vi "picoquant_initialize_acq_mode.vi"(8 "error in (no error)":errorcluster, 11 "hydraharp in":refnum<class "hydraharp.lvclass">) -> (0 "error out":errorcluster, 3 "hydraharp out":refnum<class "hydraharp.lvclass">)   [LabVIEW 2015, in "hydraharp.lvclass"]
uses:
  hydraharp.lvclass
  hydraharp.lvclass/hydraharp.ctl
  hhlib.dll
panel:
  out "version":u8[](array[numeric])
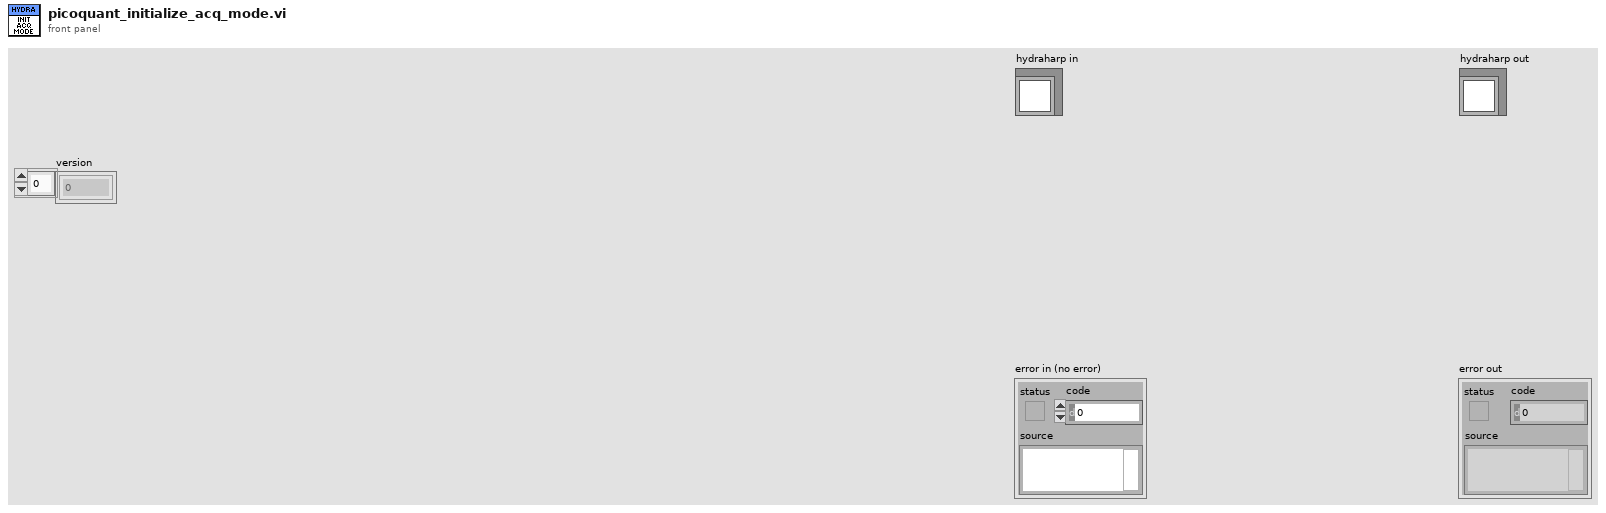
[diagram p1: front panel]
types:
  T1 = typedef "hpanel_acq_modes.ctl" = u16
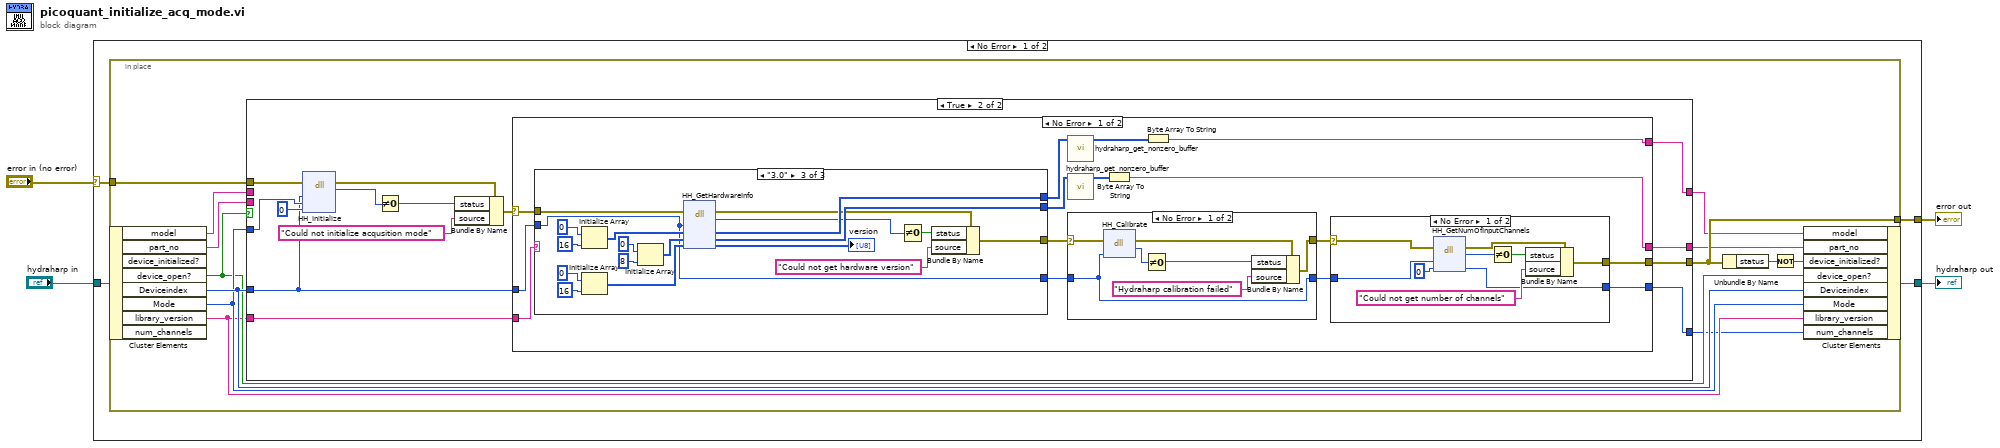
[diagram p0: block diagram]
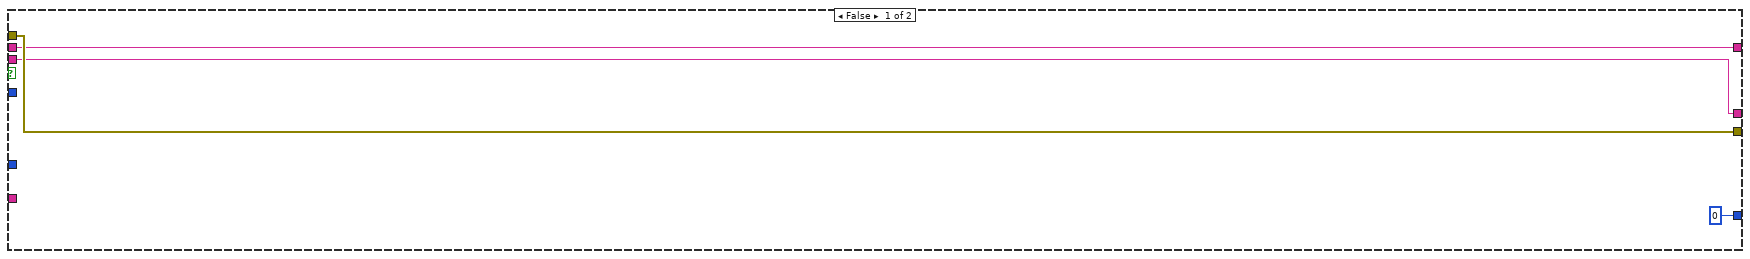
[diagram p2: hidden frame]
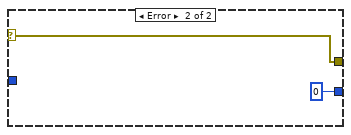
[diagram p3: hidden frame]
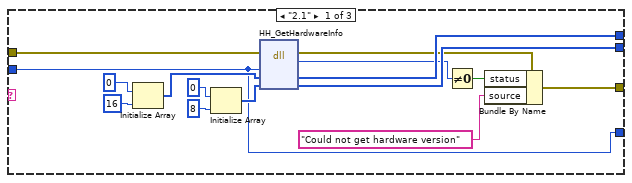
[diagram p5: hidden frame]
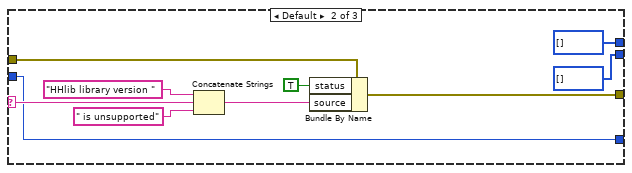
[diagram p6: hidden frame]
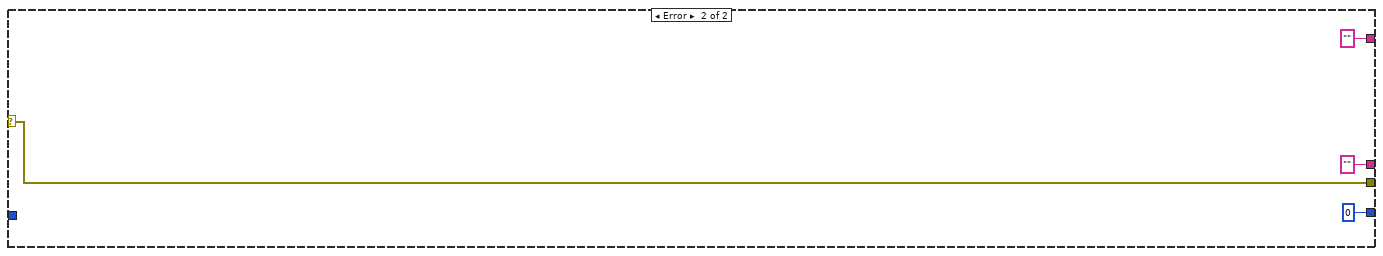
[diagram p7: hidden frame]
diagram:
  n1 = case shown="No Error" "error in (no error)" {
    selector: "error in (no error)" -> [w7 w124]
    tunnel: [w6 w124] -> w1
    tunnel: [w5 w123] -> w2
    tunnel: "hydraharp in" -> [w8 w123]
    frame No Error {
      n2 = in-place {
        in-place-border: w7 -> [w21]
        in-place-border: [w17] -> w6
        n3 = in-place-cluster #1(w8) -> ("model"=w12:string, "part_no"=w11:string, "device_open?"=w18:bool, "Deviceindex"=w20:i32, "Mode"=w19:T1, "library_version"=w10:string)  [unwired: 2 out]
        n4 = case shown="True" w18 {
          tunnel: w21 -> [w25 w39]
          tunnel: [w25 w36] -> w17
          tunnel: w20 -> [_ w35]
          tunnel: w19 -> [_ w37]
          tunnel: [w24 w34] -> w14
          tunnel: [w23 w33] -> w13
          tunnel: w12 -> [w24 _]
          tunnel: w11 -> [w23 _]
          tunnel: w10 -> [_ w32]
          tunnel: [0 ("num_channels") w26] -> w9
          frame False {
          }
          frame True {
            n5 = dll-call lib="hhlib.dll" fn="HH_Initialize"(error in=w39, "devidx"=w35, "mode"=w37, "refsrc"=0) -> (error out=w30:errorcluster, w31:i32)  [unwired: 5 in, 1 out]
            n6 = Not Equal To 0?(x=w31) -> (x != 0?=w29:bool)
            n7 = Bundle By Name(cluster=w30, "status"=w29, "source"="Could not initialize acqusition mode") -> (w27:errorcluster)
            n8 = case shown="No Error" w27 {
              selector: w27 -> [w44 w120]
              tunnel: [w42 w120] -> w36
              tunnel: w35 -> [w54 _]
              tunnel: [w48 "" ("string")] -> w34
              tunnel: [w47 "" ("string")] -> w33
              tunnel: w32 -> [w46 _]
              tunnel: [w40 0 ("num_channels")] -> w26
              frame No Error {
                n9 = case shown="\"3.0\"" w46 {
                  selector: w46 -> [_ w96 _]
                  tunnel: w44 -> [w89 w94 w118]
                  tunnel: w54 -> [w80 w90 w105]
                  tunnel: [w77 w93 w100] -> w53
                  tunnel: [w82 u8[] [] ("Model") w111] -> w52
                  tunnel: [w81 u8[] [] ("Partno") w110] -> w51
                  tunnel: [w80 w90 w105] -> w45
                  frame "2.1" {
                    n10 = Initialize Array(u8 0 ("element"), 16 ("dimension size")) -> (w86:u8[])
                    n11 = Initialize Array(u8 0 ("element"), 8 ("dimension size")) -> (w83:u8[])
                    n12 = dll-call lib="hhlib.dll" fn="HH_GetHardwareInfo" label="HH_GetHardwareVersion"(error in=w89, "devidx"=w80, "Model"=w86, "Partno"=w83) -> (error out=w78:errorcluster, "return type"=w76:i32, "Model"=w82:u8[], "Partno"=w81:u8[])  [unwired: 3 in, 1 out]
                    n13 = Not Equal To 0?(x=w76) -> (x != 0?=w75:bool)
                    n14 = Bundle By Name(cluster=w78, "status"=w75, "source"="Could not get hardware version") -> (w77:errorcluster)
                  }
                  frame Default {
                    n15 = Concatenate Strings("HHlib library version " ("string"), w96, " is unsupported" ("string")) -> (w91:string)
                    n16 = Bundle By Name(cluster=w94, "status"=TRUE, "source"=w91) -> (w93:errorcluster)
                  }
                  frame "3.0" {
                    n17 = Initialize Array(u8 0 ("element"), 16 ("dimension size")) -> (w115:u8[])
                    n18 = Initialize Array(u8 0 ("element"), 16 ("dimension size")) -> (w107:u8[])
                    n19 = Initialize Array(u8 0 ("element"), 8 ("dimension size")) -> (w112:u8[])
                    n20 = dll-call lib="hhlib.dll" fn="HH_GetHardwareInfo" label="HH_GetHardwareVersion"(error in=w118, "devidx"=w105, "Model"=w115, "Partno"=w112, "version"=w107) -> (error out=w103:errorcluster, "return type"=w104:i32, "Model"=w111:u8[], "Partno"=w110:u8[], "version"=→"version":u8[])  [unwired: 3 in, 1 out]
                    n21 = Not Equal To 0?(x=w104) -> (x != 0?=w102:bool)
                    n22 = Bundle By Name(cluster=w103, "status"=w102, "source"="Could not get hardware version") -> (w100:errorcluster)
                  }
                }
                n23 = call "hydraharp_get_nonzero_buffer.vi"("buffer"=w52) -> ("subarray"=w49:u8[])  [unwired: 10 in]
                n24 = call "hydraharp_get_nonzero_buffer.vi"("buffer"=w51) -> ("subarray"=w50:u8[])  [unwired: 10 in]
                n25 = case shown="No Error" w53 {
                  selector: w53 -> [w72 w74]
                  tunnel: w45 -> [w66 w73]
                  tunnel: [w69 w74] -> w43
                  tunnel: [w66 w73] -> w41
                  frame No Error {
                    n26 = dll-call lib="hhlib.dll" fn="HH_Calibrate"(error in=w72, "devidx"=w66) -> (error out=w70:errorcluster, "return type"=w71:i32)  [unwired: 3 in, 1 out]
                    n27 = Not Equal To 0?(x=w71) -> (x != 0?=w68:bool)
                    n28 = Bundle By Name(cluster=w70, "status"=w68, "source"="Hydraharp calibration failed") -> (w69:errorcluster)
                  }
                  frame Error {
                  }
                }
                n29 = Byte Array To String(unsigned byte array=w50) -> (string=w47:string)
                n30 = Byte Array To String(unsigned byte array=w49) -> (string=w48:string)
                n31 = case shown="No Error" w43 {
                  selector: w43 -> [w62 w65]
                  tunnel: [w57 w65] -> w42
                  tunnel: w41 -> [w63 _]
                  tunnel: [w55 0 ("num_channels")] -> w40
                  frame No Error {
                    n32 = dll-call lib="hhlib.dll" fn="HH_GetNumOfInputChannels"(error in=w62, "devidx"=w63, "num_channels"=0) -> (error out=w60:errorcluster, "return type"=w61:i32, "num_channels"=w55:i32)  [unwired: 3 in, 1 out]
                    n33 = Not Equal To 0?(x=w61) -> (x != 0?=w59:bool)
                    n34 = Bundle By Name(cluster=w60, "status"=w59, "source"="Could not get number of channels") -> (w57:errorcluster)
                  }
                  frame Error {
                  }
                }
              }
              frame Error {
              }
            }
          }
        }
        n35 = Unbundle By Name(w17) -> ("status"=w16:bool)
        n36 = Not(x=w16) -> (.not. x?=w15:bool)
        n37 = in-place-cluster #1("model"=w14, "part_no"=w13, "device_initialized?"=w15, "device_open?"=w18, "Deviceindex"=w20, "Mode"=w19, "library_version"=w10, "num_channels"=w9) -> (w5:refnum<class "hydraharp.lvclass">)
      }
    }
    frame Error {
    }
  }
  "error out" <- w1
  "hydraharp out" <- w2
